vi "Create FileTx Notification.vi"(8 "error in (no error)":errorcluster, 11 "FTP in":refnum<class "FTP.lvclass">) -> (0 "error out":errorcluster, 3 "FTP out":refnum<class "FTP.lvclass">)   [LabVIEW 2017, in "FTP_UpgradeCSMF.lvlib" / "FTP.lvclass"]
uses:
  FTP.lvclass
  controls/File Transfer Status.ctl
  FTP.lvclass/FTP.ctl
panel:
  in  "File Transfer Status":T1
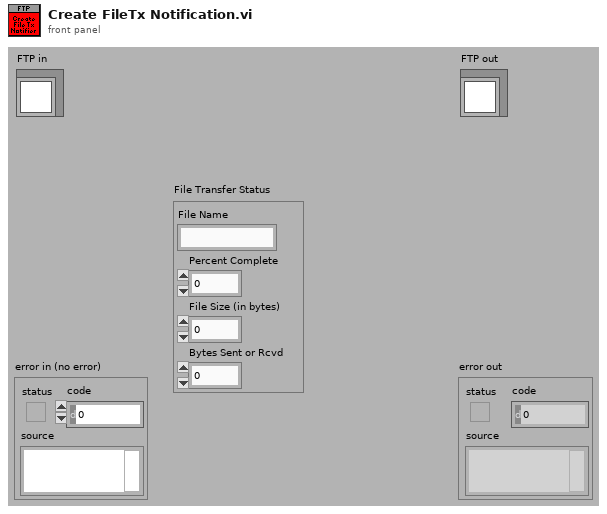
[diagram p1: front panel]
types:
  T1 = typedef "FTP_UpgradeCSMF.lvlib/FTP.lvclass/File Transfer Status.ctl" = cluster{"File Name":string, "Percent Complete":u8, "File Size (in bytes)":i64, "Bytes Sent or Rcvd":i64}
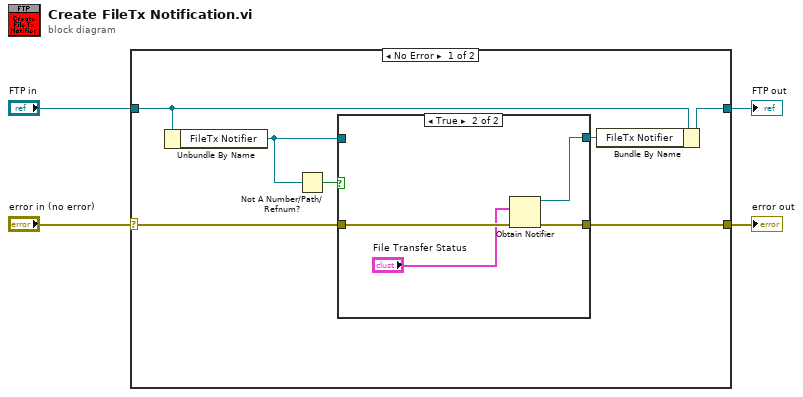
[diagram p0: block diagram]
diagram:
  n1 = case shown="No Error" "error in (no error)" {
    selector: "error in (no error)" -> [w11 w19]
    tunnel: [w10 w19] -> w3
    tunnel: [w9 w18] -> w1
    tunnel: "FTP in" -> [w7 w18]
    frame No Error {
      n2 = Unbundle By Name(w7) -> ("FileTx Notifier"=w5:refnum<notifier>)
      n3 = Not A Number/Path/Refnum?(number/path/refnum=w5) -> (NaN/Path/Refnum?=w6:bool)
      n4 = case shown="True" w6 {
        tunnel: w11 -> [w12 w17]
        tunnel: [w12 w16] -> w10
        tunnel: [w13 w14] -> w8
        tunnel: w5 -> [w13 _]
        frame False {
        }
        frame True {
          n5 = Obtain Notifier(notification data type="File Transfer Status", error in (no error)=w17) -> (notifier out=w14:refnum<notifier>, error out=w16:errorcluster)  [unwired: 2 in, 1 out]
        }
      }
      n6 = Bundle By Name(cluster=w7, "FileTx Notifier"=w8) -> (w9:refnum<class "FTP.lvclass">)
    }
    frame Error {
    }
  }
  "error out" <- w3
  "FTP out" <- w1
